vi "setDIO.vi"(8 "error in (no error)":errorcluster, 11 "DIO state":T1) -> (0 "error out":errorcluster)   [LabVIEW 2010, in "TPVG_DLL.lvlib"]
doc: "get DIO config information and state\n------------------------------------------\nAuthor: Dang Lam\nEmail: danglamtd@gmail.com"
uses:
  TPVG_DLL.lvlib
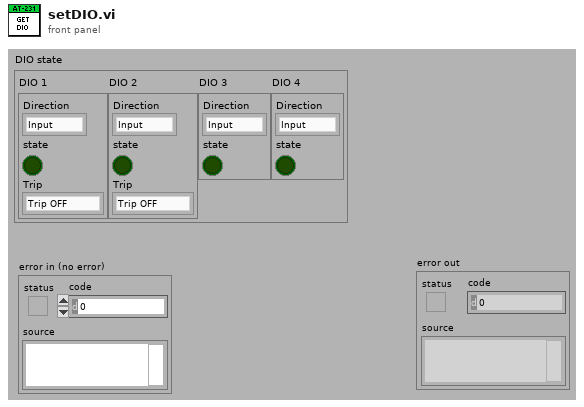
[diagram p1: front panel]
types:
  T1 = cluster{"DIO 1":cluster{"Direction":enum16{"Input", "Output"}, "state":bool, "Trip":enum16{"Trip OFF", "Trip ON"}}, "DIO 2":cluster{"Direction":enum16{"Input", "Output"}, "state":bool, "Trip":enum16{"Trip OFF", "Trip ON"}}, "DIO 3":cluster{"Direction":enum16{"Input", "Output"}, "state":bool}, "DIO 4":cluster{"Direction":enum16{"Input", "Output"}, "state":bool}}
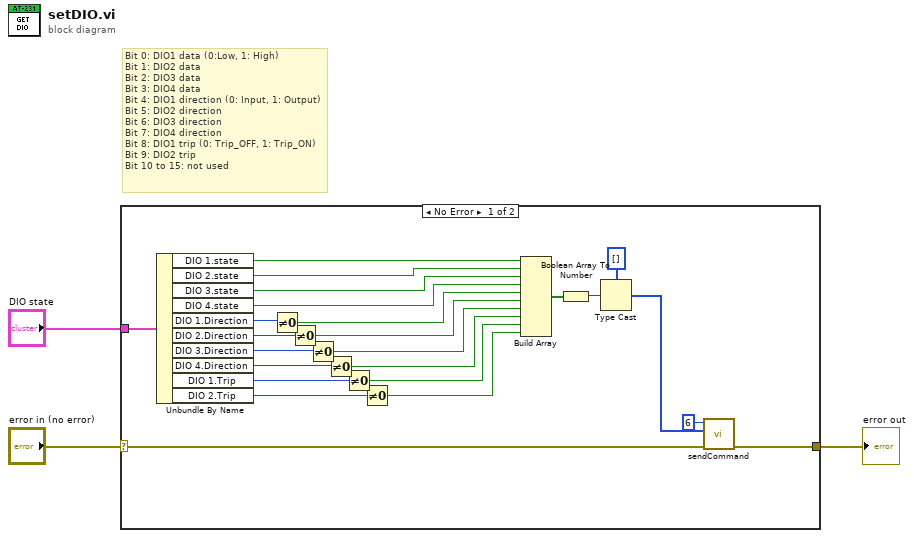
[diagram p0: block diagram]
diagram:
  # "Bit 0: DIO1 data (0:Low, 1: High)\nBit 1: DIO2 data\nBit 2: DIO3 data\nBit 3: DIO4 data\nBit 4: DIO1 direction (0: Input, 1: Output)\nBit 5: DIO2 direction\nBit 6: DIO3 direction\nBit 7: DIO4 direction\nBit 8: DIO1 trip (0: Trip_OFF, 1: Trip_ON)\nBit 9: DIO2 trip\nBit 10 to 15: not used"
  n1 = case shown="No Error" "error in (no error)" {
    selector: "error in (no error)" -> [w9 w28]
    tunnel: [w8 w28] -> w2
    tunnel: "DIO state" -> [w27 _]
    frame No Error {
      n2 = Unbundle By Name(w27) -> ("DIO 1.state"=w20:bool, "DIO 2.state"=w19:bool, "DIO 3.state"=w18:bool, "DIO 4.state"=w17:bool, "DIO 1.Direction"=w26:enum16{"Input", "Output"}, "DIO 2.Direction"=w25:enum16{"Input", "Output"}, "DIO 3.Direction"=w24:enum16{"Input", "Output"}, "DIO 4.Direction"=w23:enum16{"Input", "Output"}, "DIO 1.Trip"=w22:enum16{"Trip OFF", "Trip ON"}, "DIO 2.Trip"=w21:enum16{"Trip OFF", "Trip ON"})
      n3 = Not Equal To 0?(x=w26) -> (x != 0?=w16:bool)
      n4 = Not Equal To 0?(x=w25) -> (x != 0?=w15:bool)
      n5 = Not Equal To 0?(x=w24) -> (x != 0?=w14:bool)
      n6 = Not Equal To 0?(x=w23) -> (x != 0?=w13:bool)
      n7 = Not Equal To 0?(x=w22) -> (x != 0?=w12:bool)
      n8 = Not Equal To 0?(x=w21) -> (x != 0?=w11:bool)
      n9 = Build Array(w20, w19, w18, w17, w16, w15, w14, w13, w12, w11) -> (w10:bool[])
      n10 = Boolean Array To Number(Boolean array=w10) -> (number=w6:u16)
      n11 = Type Cast(type=u8[] [], x=w6) -> (*(type *) &x=w4:u8[])
      n12 = call "sendCommand.vi"("error in (no error)"=w9, "Data in"=w4, "Command ID"=u16 6) -> ("error out"=w8:errorcluster)  [unwired: 7 in, 1 out]
    }
    frame Error {
    }
  }
  "error out" <- w2
